vi "(SubVI).vi"(6 "Sampling Frequency":dbl, 9 "Carrier Frequency":dbl, 10 "Data Frequency":dbl, 11 "Iterations":i32) -> (1 "Modulated Signal":dbl[](graph), 2 "Modulating Square":i16[](graph), 3 "Modulating Sin":dbl[](graph), 4 "Carrier Signal":dbl[](graph))   [LabVIEW 2015]
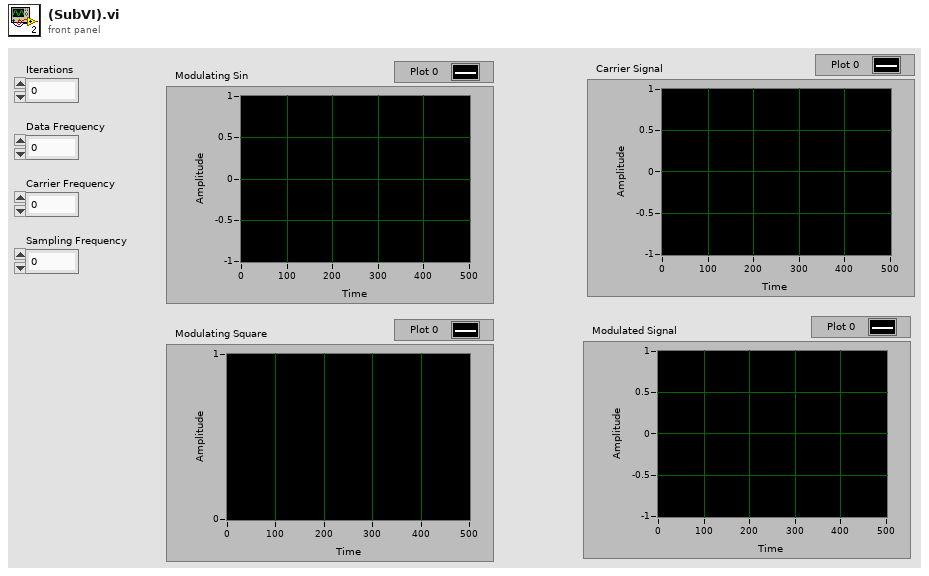
[diagram p1: front panel]
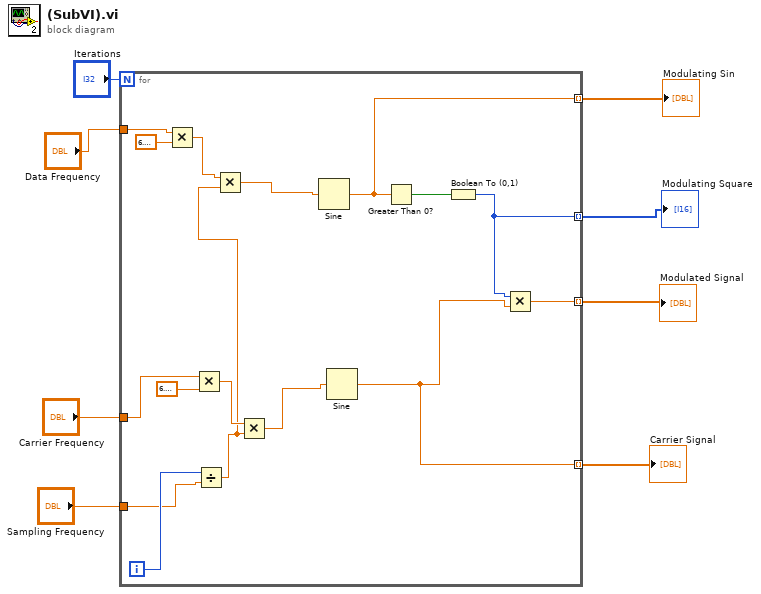
[diagram p0: block diagram]
diagram:
  n1 = for {
    N: "Iterations" -> [_]
    tunnel: "Sampling Frequency" -> [w23]
    tunnel: "Carrier Frequency" -> [w22]
    tunnel: "Data Frequency" -> [w17]
    tunnel: [w12] -> w5 mode=indexing
    tunnel: [w11] -> w6 mode=indexing
    tunnel: [w10] -> w7 mode=indexing
    tunnel: [w9] -> w8 mode=indexing
    i -> [w24]
    n2 = Multiply(x=w17, y=6.283185307179586) -> (x*y=w16:dbl)
    n3 = Multiply(x=w22, y=6.283185307179586) -> (x*y=w20:dbl)
    n4 = Divide(x=w24, y=w23) -> (x/y=w15:dbl)
    n5 = Multiply(x=w16, y=w15) -> (x*y=w14:dbl)
    n6 = Multiply(x=w20, y=w15) -> (x*y=w19:dbl)
    n7 = Sine(x=w14) -> (sin(x)=w10:dbl)
    n8 = Sine(x=w19) -> (sin(x)=w9:dbl)
    n9 = Greater Than 0?(x=w10) -> (x > 0?=w13:bool)
    n10 = Boolean To (0,1)(Boolean=w13) -> (0, 1=w11:i16)
    n11 = Multiply(x=w11, y=w9) -> (x*y=w12:dbl)
  }
  "Modulated Signal" <- w5
  "Modulating Square" <- w6
  "Modulating Sin" <- w7
  "Carrier Signal" <- w8
